vi "CMI ckd2 Get Clock Source.vi"(8 "error in":errorcluster, 11 "session":T2) -> (0 "error out":errorcluster, 1 "active clock source":T1, 2 "selected clock source":T1, 3 "session out":T2)   [LabVIEW 2020, in "AWG.lvlib"]
doc: "Gets clock source of the clock divider. Returns selection and actually active mode."
uses:
  AWG.lvlib
  CMI ckd2 Session.ctl
  CMI ckd2 Source Mode.ctl
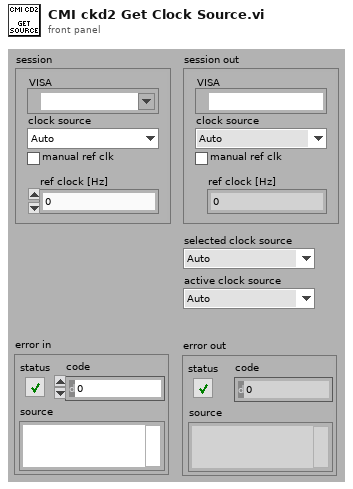
[diagram p1: front panel]
types:
  T1 = typedef "AWG.lvlib/CMI ckd2 Source Mode.ctl" = enum16{"Auto", "LF clock", "HF clock", "Internal"}
  T2 = typedef "AWG.lvlib/CMI ckd2 Session.ctl" = cluster{"VISA":refnum<visa-resource-name>, "clock source":T1, "manual ref clk":bool, "ref clock [Hz]":dbl}
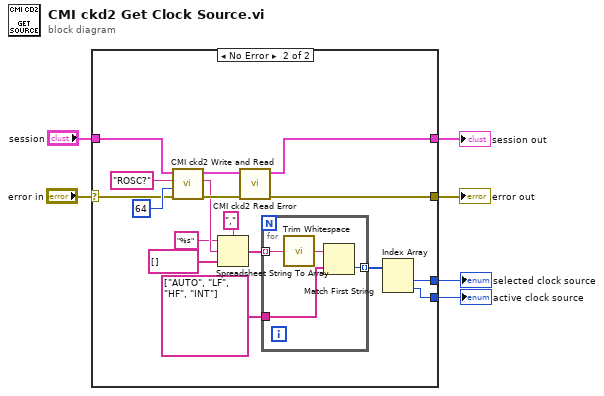
[diagram p0: block diagram]
diagram:
  n1 = case shown="No Error" "error in" {
    selector: "error in" -> [w7 w18]
    tunnel: [w8 w22] -> w4
    tunnel: [w7 w21] -> w6
    tunnel: "session" -> [w8 w25]
    tunnel: [_ w11] -> w2
    tunnel: [_ w10] -> w1
    frame Error {
    }
    frame No Error {
      n2 = call "CMI ckd2 Write and Read.vi"("error in"=w18, "read byte count (0 - no receive)"=u32 64, "command"="ROSC?" ("format string"), "session"=w25) -> ("error out"=w24:errorcluster, "read buffer"=w17:string, "session out"=w23:T2)  [unwired: 5 in]
      n3 = Spreadsheet String To Array(delimiter (Tab)=",", format string="%s", spreadsheet string=w17, array type (2D Dbl)=string[] []) -> (array=w14:string[])
      n4 = call "CMI ckd2 Read Error.vi"("error in"=w24, "session"=w23) -> ("error out"=w21:errorcluster, "session out"=w22:T2)  [unwired: 7 in, 1 out]
      n5 = for {
        tunnel: w14 -> [w29] mode=indexing
        tunnel: string[] ["AUTO", "LF", "HF", "INT"] -> [w28]
        tunnel: [w27] -> w12 mode=indexing
        n6 = call <vilib>:"Trim Whitespace.vi"("string"=w29) -> ("trimmed string"=w26:string)  [unwired: 1 in]
        n7 = Match First String(2:w28, 3:w26) -> (0:w27:i32)  [unwired: 1 out]
      }
      n8 = Index Array(array=w12) -> (element #1=w11:i32, element #2=w10:i32)  [unwired: 2 in]
    }
  }
  "error out" <- w6
  "session out" <- w4
  "selected clock source" <- w2
  "active clock source" <- w1
